vi "run.vi"   [LabVIEW 2016, in "LineFollower2Sensor.lvrbt"]
uses:
  LineFollower2Sensor.lvrbt
  <vilib>/NXT/Hardware/Plugins/Tetrix DC Motor/TetrixDCMotorAddress.ctl
  <vilib>/NXT/Block Support/NXT_InputPort.ctl
  <vilib>/NXT/Dual Mode Library/Sensors/EV3_Color_Reflect.vi
  <vilib>/NXT/NXTIO Xnodes/NXTIONodeSubVIs/TETRIX IO Move DC Motors.vi
  <vilib>/NXT/Subs/LVHSConnector.ctl
  <vilib>/NXT/NXTIO Xnodes/AddressXNode/NXTIOAddress.xnode
  <vilib>/NXT/NXTIO Xnodes/NXTIOXNode/NXTIO.xnode
  <vilib>/NXT/LegoClasses/BrickReference/BrickReference.lvclass
types:
  T1 = typedef "TetrixDCMotorAddress.ctl" = i32
  T2 = cluster{"TetrixDCMotor":T1, "TetrixDCMotor 2":T1}
  T3 = typedef "NXT_InputPort.ctl" = u32
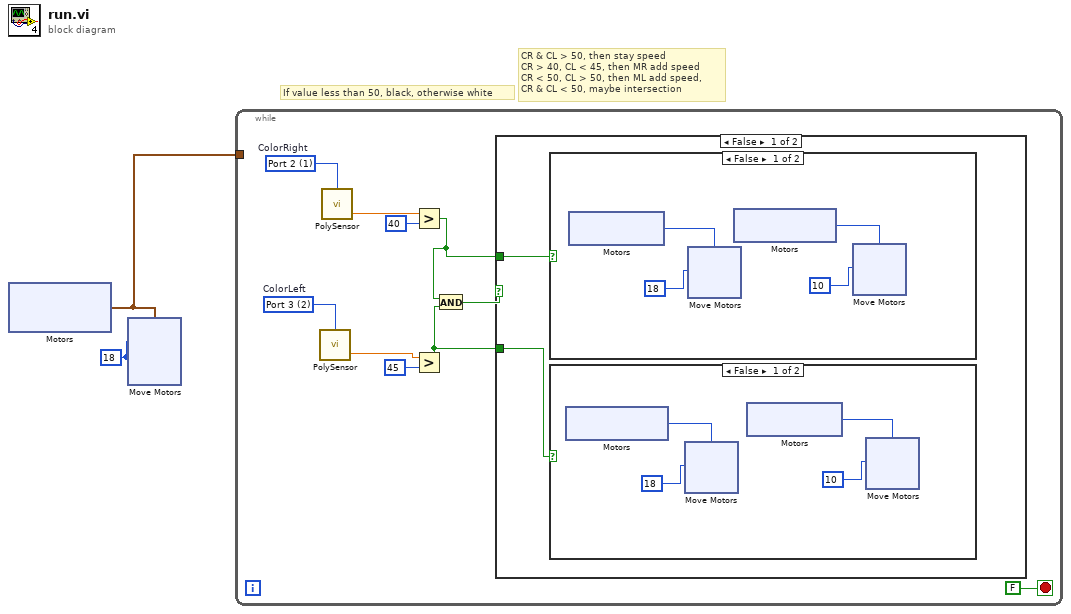
[diagram p0: block diagram]
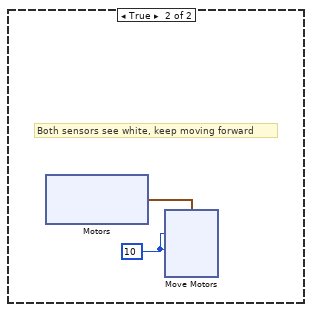
[diagram p4: hidden frame]
diagram:
  w2 = i8 18 ("Power/Speed 2")
  # "CR & CL > 50, then stay speed\nCR > 40, CL < 45, then MR add speed\nCR < 50, CL > 50, then ML add speed,\nCR & CL < 50, maybe intersection"
  # "If value less than 50, black, otherwise white"
  n1 = xnode "Motors"() -> ("Motor"=w1:cluster{"TetrixDCMotor":T1, "TetrixDCMotor":T1})
  n2 = xnode "Move Motors"("Power/Speed 2"=w2, "Power/Speed 1"=w2, "Motors"=w1) -> ()  [unwired: 1 in, 1 out]
  n3 = while {
    tunnel: w1 -> [_]
    stop <- FALSE stop-if-true
    w10 = T3 2 items=["Port 1", "Port 2", "Port 3", "Port 4"]  # ColorLeft
    w11 = T3 1 items=["Port 1", "Port 2", "Port 3", "Port 4"]  # ColorRight
    n4 = call-poly <vilib>:"PolySensor.vi"("Port (Port 1)"=w10) -> ("Scaled Value"=w6:sgl)  [unwired: 2 in, 1 out]
    n5 = call-poly <vilib>:"PolySensor.vi"("Port (Port 1)"=w11) -> ("Scaled Value"=w9:sgl)  [unwired: 2 in, 1 out]
    n6 = Greater?(x=w9, y=i16 40) -> (0:w4:bool)
    n7 = Greater?(x=w6, y=i16 45) -> (0:w3:bool)
    n8 = And(x=w4, y=w3) -> (x .and. y?=w5:bool)
    n9 = case "Case 1 and 4" shown="False" w5 {
      tunnel: w4 -> [w14 _]
      tunnel: w3 -> [w13 _]
      frame False {
        n10 = case shown="False" w14 {
          frame False {
            n11 = xnode "Motors"() -> ("Motor"=w37:T1)
            n12 = xnode "Move Motors"("Power/Speed 1"=i8 18 ("Power/Speed 2"), "Motors"=w37) -> ()  [unwired: 1 in, 1 out]
            n13 = xnode "Motors"() -> ("Motor"=w35:T1)
            n14 = xnode "Move Motors"("Power/Speed 1"=i8 10 ("Power/Speed 2"), "Motors"=w35) -> ()  [unwired: 1 in, 1 out]
          }
          frame True {
          }
        }
        n15 = case shown="False" w13 {
          frame False {
            n16 = xnode "Motors"() -> ("Motor"=w18:T1)
            n17 = xnode "Move Motors"("Power/Speed 1"=i8 18 ("Power/Speed 2"), "Motors"=w18) -> ()  [unwired: 1 in, 1 out]
            n18 = xnode "Motors"() -> ("Motor"=w16:T1)
            n19 = xnode "Move Motors"("Power/Speed 1"=i8 10 ("Power/Speed 2"), "Motors"=w16) -> ()  [unwired: 1 in, 1 out]
          }
          frame True {
          }
        }
      }
      frame True {
        w55 = i8 10 ("Power/Speed 2")
        # "Both sensors see white, keep moving forward"
        n20 = xnode "Motors"() -> ("Motor"=w56:cluster{"TetrixDCMotor":T1, "TetrixDCMotor":T1})
        n21 = xnode "Move Motors"("Power/Speed 2"=w55, "Power/Speed 1"=w55, "Motors"=w56) -> ()  [unwired: 1 in, 1 out]
      }
    }
  }
